vi "Read Database.vi"(8 "error in (no error)":errorcluster, 11 "Table Configuration Adv Schema DB in":refnum<class "Table Configuration Adv Schema DB.lvclass">) -> (0 "error out":errorcluster, 2 "Database":refnum<class "Database Adv Schema.lvclass">, 3 "Table Configuration Adv Schema DB out":refnum<class "Table Configuration Adv Schema DB.lvclass">)   [LabVIEW 2020]
uses:
  Table Configuration Adv Schema DB.lvclass
  C:/Users/User/Desktop/Raman Program/Database OOP/source/Database OOP/Table Libraries/Basic Table/Configuration/Table Configuration Class/Table Configuration.lvclass
  C:/Users/User/Desktop/Raman Program/Database OOP/source/Database OOP/Table Libraries/Table Configuration Interface/Table Configuration Interface.lvclass
  C:/Users/User/Desktop/Raman Program/Database OOP/source/Database OOP/Table Libraries/Basic Table/Configuration/Table Configuration Adv Schema DB/Table Configuration Adv Schema DB.lvclass
  Database Libraries/Database Interfaces/Database Advanced Schema Class/Database Adv Schema.lvclass
  C:/Users/User/Desktop/Raman Program/Database OOP/source/Database OOP/Database Libraries/Database Interfaces/Database Advanced Schema Class/Database Adv Schema.lvclass
  C:/Users/User/Desktop/Raman Program/Database OOP/source/Database OOP/Database Libraries/Database Interfaces/Database Interface Class/Database Interface.lvclass
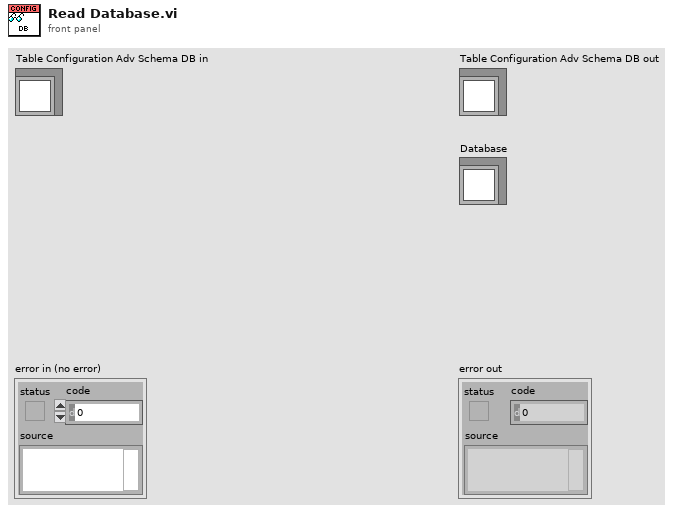
[diagram p1: front panel]
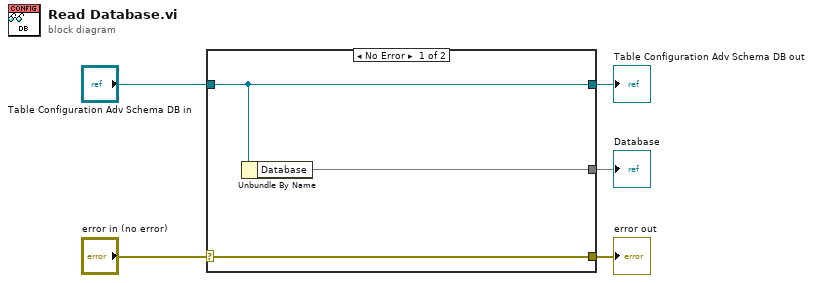
[diagram p0: block diagram]
diagram:
  n1 = case shown="No Error" "error in (no error)" {
    selector: "error in (no error)" -> [w8 w9]
    tunnel: [w8 w9] -> w4
    tunnel: [w7 w10] -> w2
    tunnel: "Table Configuration Adv Schema DB in" -> [w7 w10]
    tunnel: [w6 _] -> w1
    frame No Error {
      n2 = Unbundle By Name(w7) -> ("Database"=w6)
    }
    frame Error {
    }
  }
  "error out" <- w4
  "Table Configuration Adv Schema DB out" <- w2
  "Database" <- w1
